vi "ATE_Settings.vi"(9 "Variable to Read":string[](array[string]), 10 "file name":string="ATE_settings.txt" caption="default name", 11 "start path":path=path "Z:/Data 2/ATE_labVIEW_code") -> (0 "error out":errorcluster, 3 "NewVariables":cluster{"Name":string, "Value":dbl}[](array[cluster]))   [LabVIEW 2009]
panel:
  out "ATE Settings":string[](array[string])
  out "FILE":path caption="selected path"
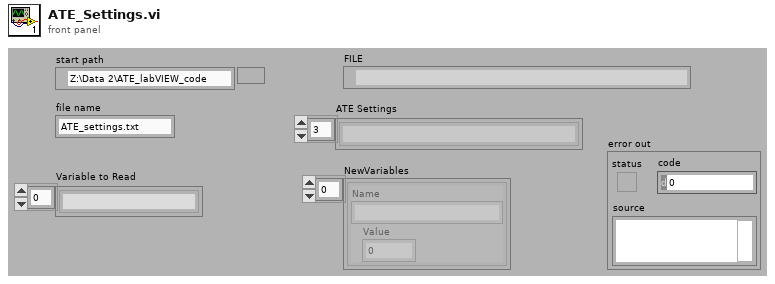
[diagram p1: front panel]
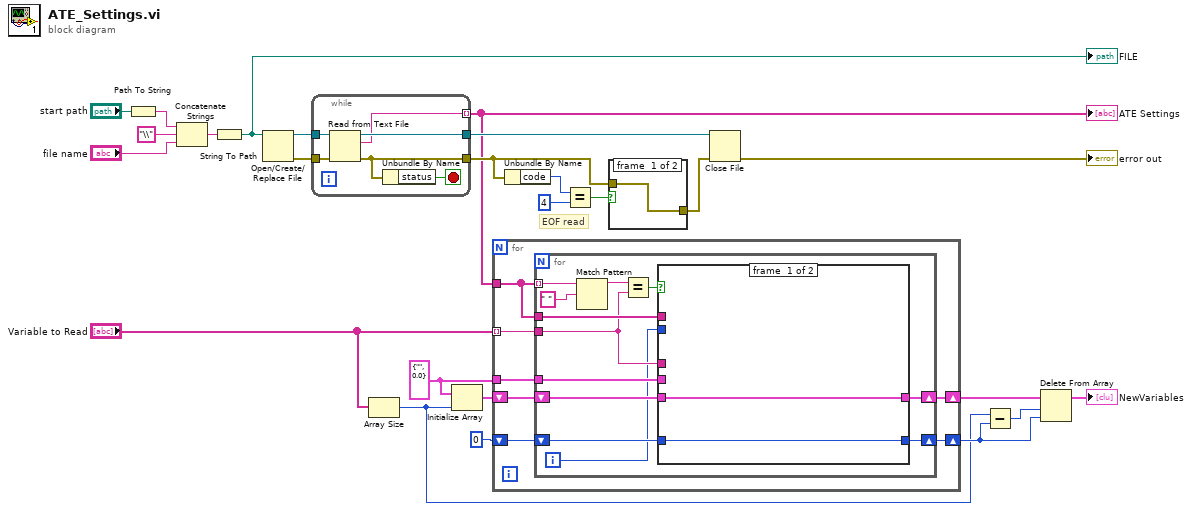
[diagram p0: block diagram]
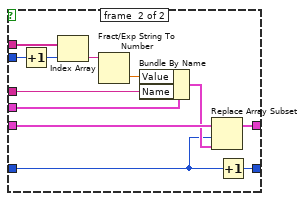
[diagram p2: hidden frame]
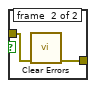
[diagram p3: hidden frame]
diagram:
  w8 = cluster{"Name":string, "Value":dbl} {"Name"="", "Value"=0.0} ("Variable")
  # "EOF read"
  n1 = Path To String(path="start path") -> (string=w24:string)
  n2 = Concatenate Strings(w24, "\\" ("string"), "file name") -> (w21:string)
  n3 = String To Path(string=w21) -> (path=w20:path)
  "FILE" <- w20
  n4 = Open/Create/Replace File(file path (use dialog)=w20) -> (refnum out=w18:refnum<file>, error out=w17:errorcluster)  [unwired: 5 in, 1 out]
  n5 = while {
    tunnel: w18 -> [w31]
    tunnel: w17 -> [w30]
    tunnel: [w29] -> w16
    tunnel: [w27] -> w12
    tunnel: [w28] -> w10 mode=indexing
    stop <- w26 stop-if-true
    n6 = Read from Text File(file (use dialog)=w31, error in=w30) -> (refnum out=w29:refnum<file>, text=w28:string, error out=w27:errorcluster)  [unwired: 2 in, 1 out]
    n7 = Unbundle By Name(w27) -> ("status"=w26:bool)
  }
  "ATE Settings" <- w10
  n8 = Array Size(array="Variable to Read") -> (size(s)=w2:i32)
  n9 = Initialize Array(w8, w2) -> (w7:cluster{"Name":string, "Value":dbl}[])
  n10 = for {
    tunnel: w10 -> [w37]
    tunnel: "Variable to Read" -> [w38] mode=indexing
    tunnel: w8 -> [w36]
    shift-right: [w32] -> w3
    shift-left: 0 -> [w34]
    shift-right: [w33] -> w5
    shift-left: w7 -> [w35]
    n11 = for {
      tunnel: w37 -> [w43] mode=indexing
      tunnel: w38 -> [w45]
      tunnel: w37 -> [w49]
      tunnel: w36 -> [w48]
      shift-right: [w41] -> w33
      shift-left: w35 -> [w47]
      shift-right: [w40] -> w32
      shift-left: w34 -> [w46]
      i -> [w39]
      n12 = Match Pattern(string=w43, regular expression=" ") -> (before substring=w42:string)  [unwired: 1 in, 3 out]
      n13 = Equal?(x=w42, y=w45) -> (x = y?=w50:bool)
      n14 = case shown="True" w50 {
        tunnel: w49 -> [_ w64]
        tunnel: w48 -> [_ w61]
        tunnel: w45 -> [_ w59]
        tunnel: w39 -> [_ w58]
        tunnel: w47 -> [w52 w57]
        tunnel: [w52 w56] -> w41
        tunnel: w46 -> [w51 w53]
        tunnel: [w51 w55] -> w40
        frame #0 {
        }
        frame #1 {
          n15 = Increment(x=w58) -> (x+1=w63:i32)
          n16 = Index Array(array=w64, index=w63) -> (element=w62:string)
          n17 = Fract/Exp String To Number(string=w62) -> (number=w60:dbl)  [unwired: 3 in, 1 out]
          n18 = Bundle By Name(cluster=w61, "Value"=w60, "Name"=w59) -> (w54:cluster{"Name":string, "Value":dbl})
          n19 = Replace Array Subset(array=w57, new element=w54, index=w53) -> (w56:cluster{"Name":string, "Value":dbl}[])
          n20 = Increment(x=w53) -> (x+1=w55:i32)
        }
      }
    }
  }
  n21 = Unbundle By Name(w12) -> ("code"=w14:i32)
  n22 = Equal?(x=w14, y=4) -> (x = y?=w15:bool)
  n23 = case shown="True" w15 {
    tunnel: w12 -> [w65 w67]
    tunnel: [w65 w66] -> w11
    frame #0 {
    }
    frame #1 {
      n24 = call <vilib>:"Clear Errors.vi"("error in (no error)"=w67) -> ("error out"=w66:errorcluster)  [unwired: 6 in]
    }
  }
  n25 = Close File(refnum=w16, error in=w11) -> (error out=→"error out":errorcluster)  [unwired: 1 out]
  n26 = Subtract(x=w2, y=w3) -> (x-y=w4:i32)
  n27 = Delete From Array(array=w5, length=w4, index=w3) -> (array with subset deleted=→"NewVariables":cluster{"Name":string, "Value":dbl}[])  [unwired: 1 out]
